vi "filter_peaks.vi"(8 "Correlation cluster":T3, 9 "Filter peak cluster":T2, 10 "Zero out":bool, 11 "Run Mode":bool) -> (0 "Blinking":bool, 1 "status":T1(ring), 3 "Filter peak output":T2)   [LabVIEW 2015]
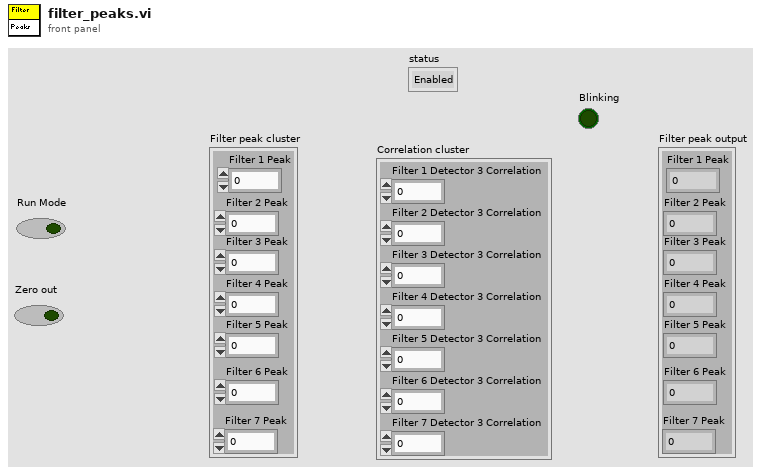
[diagram p1: front panel]
types:
  T1 = enum8{"Enabled", "Disabled", "Disabled and Grayed Out"}
  T2 = cluster{"Filter 1 Peak":i32, "Filter 2 Peak":i32, "Filter 3 Peak":i32, "Filter 4 Peak":i32, "Filter 5 Peak":i32, "Filter 6 Peak":i32, "Filter 7 Peak":i32}
  T3 = cluster{"Filter 1 Detector 3 Correlation":i32, "Filter 2 Detector 3 Correlation":i32, "Filter 3 Detector 3 Correlation":i32, "Filter 4 Detector 3 Correlation":i32, "Filter 5 Detector 3 Correlation":i32, "Filter 6 Detector 3 Correlation":i32, "Filter 7 Detector 3 Correlation":i32}
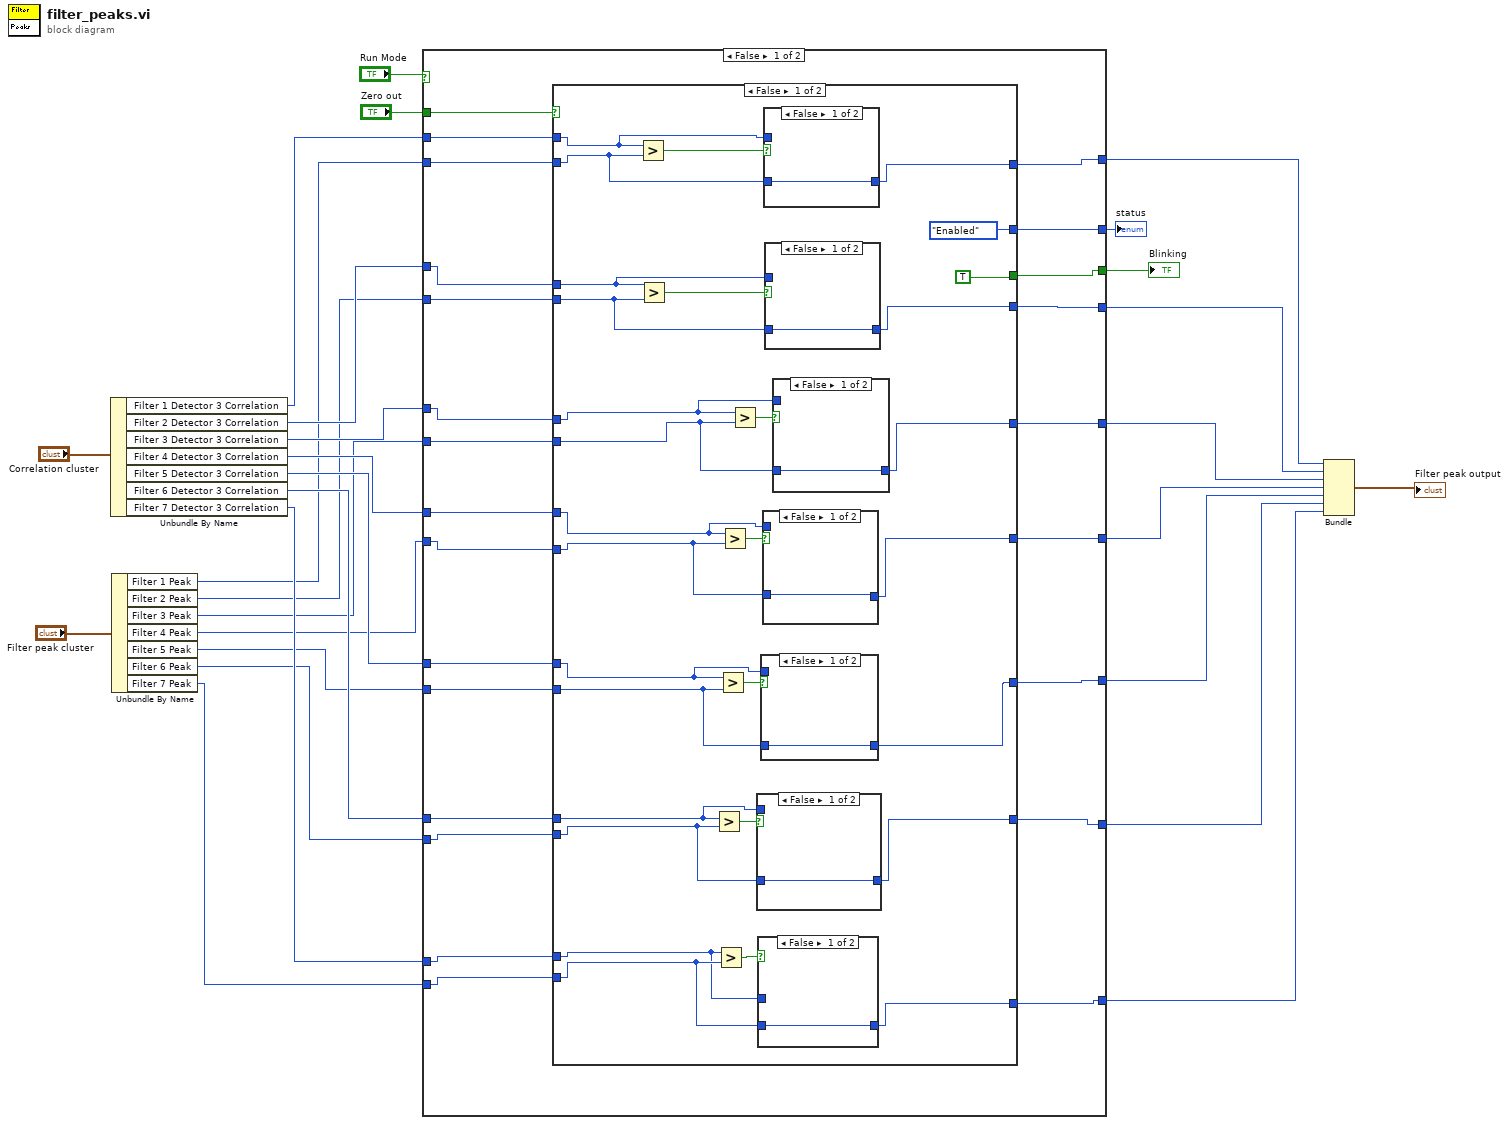
[diagram p0: block diagram]
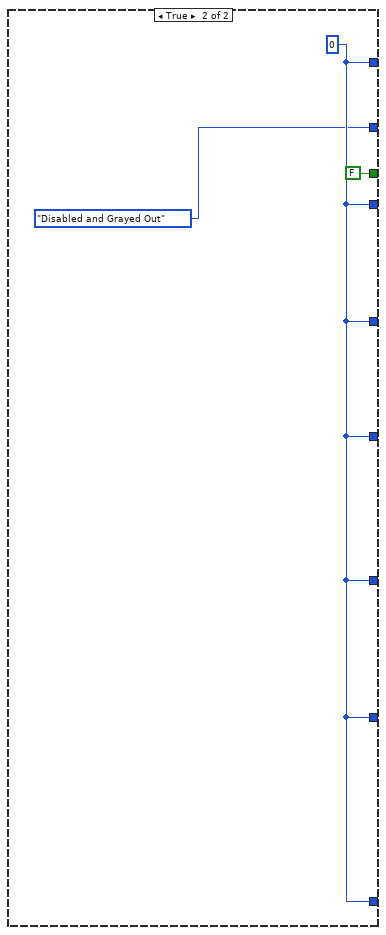
[diagram p9: hidden frame]
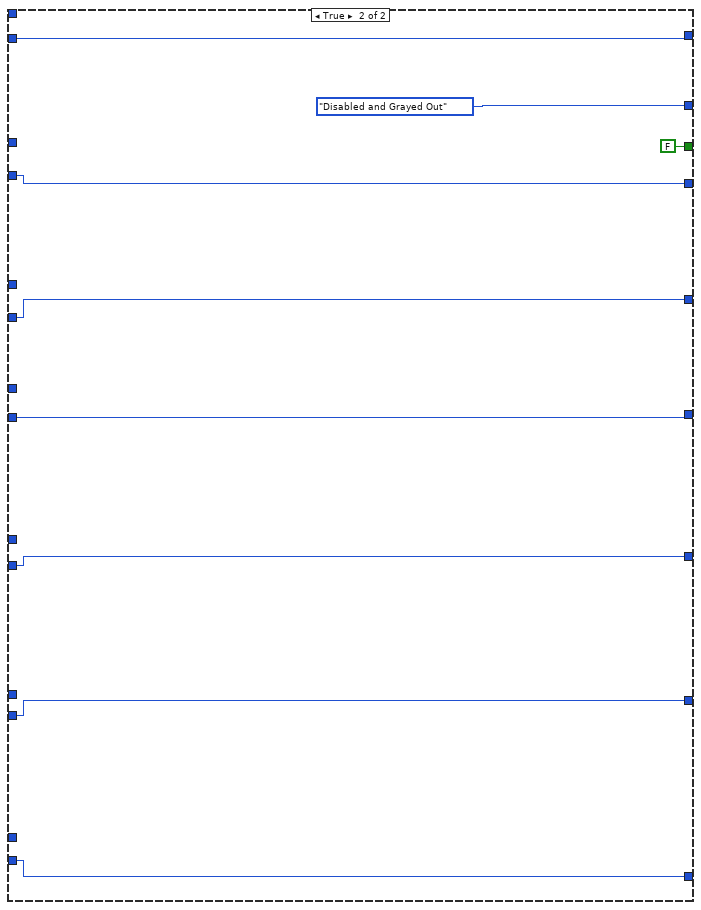
[diagram p10: hidden frame]
diagram:
  n1 = Unbundle By Name("Correlation cluster") -> ("Filter 1 Detector 3 Correlation"=w25:i32, "Filter 2 Detector 3 Correlation"=w24:i32, "Filter 3 Detector 3 Correlation"=w23:i32, "Filter 4 Detector 3 Correlation"=w22:i32, "Filter 5 Detector 3 Correlation"=w19:i32, "Filter 6 Detector 3 Correlation"=w21:i32, "Filter 7 Detector 3 Correlation"=w20:i32)
  n2 = Unbundle By Name("Filter peak cluster") -> ("Filter 1 Peak"=w17:i32, "Filter 2 Peak"=w16:i32, "Filter 3 Peak"=w15:i32, "Filter 4 Peak"=w14:i32, "Filter 5 Peak"=w13:i32, "Filter 6 Peak"=w12:i32, "Filter 7 Peak"=w11:i32)
  n3 = case shown="False" "Run Mode" {
    tunnel: [w52 w105] -> w8
    tunnel: [w51 w104] -> w7
    tunnel: [w50 w103] -> w6
    tunnel: [w49 w102] -> w5
    tunnel: [w48 w101] -> w4
    tunnel: [w47 w107] -> w10
    tunnel: [w46 w106] -> w9
    tunnel: "Zero out" -> [w45 _]
    tunnel: [w44 T1."Disabled and Grayed Out" ("Disabled")] -> w2
    tunnel: w25 -> [w43 _]
    tunnel: w24 -> [w42 _]
    tunnel: w23 -> [w41 _]
    tunnel: w22 -> [w40 _]
    tunnel: w21 -> [w38 _]
    tunnel: w20 -> [w37 _]
    tunnel: w19 -> [w39 _]
    tunnel: w17 -> [w36 w107]
    tunnel: w16 -> [w35 w106]
    tunnel: w15 -> [w34 w105]
    tunnel: w14 -> [w33 w104]
    tunnel: w13 -> [w32 w103]
    tunnel: w12 -> [w31 w102]
    tunnel: w11 -> [w30 w101]
    tunnel: [w29 FALSE] -> w1
    frame False {
      n4 = case shown="False" w45 {
        tunnel: [w67 w99] -> w52
        tunnel: [w64 w99] -> w51
        tunnel: [w61 w99] -> w50
        tunnel: [w58 w99] -> w49
        tunnel: [w55 w99] -> w48
        tunnel: [w72 w99] -> w47
        tunnel: [w70 w99] -> w46
        tunnel: [T1."Enabled" ("Disabled") T1."Disabled and Grayed Out" ("Disabled")] -> w44
        tunnel: w43 -> [w73 _]
        tunnel: w42 -> [w69 _]
        tunnel: w41 -> [w66 _]
        tunnel: w40 -> [w63 _]
        tunnel: w39 -> [w60 _]
        tunnel: w38 -> [w57 _]
        tunnel: w37 -> [w54 _]
        tunnel: w36 -> [w74 _]
        tunnel: w35 -> [w71 _]
        tunnel: w34 -> [w68 _]
        tunnel: w33 -> [w65 _]
        tunnel: w32 -> [w62 _]
        tunnel: w31 -> [w59 _]
        tunnel: w30 -> [w56 _]
        tunnel: [TRUE FALSE] -> w29
        frame False {
          n5 = Greater?(x=w73, y=w74) -> (0:w77:bool)
          n6 = Greater?(x=w69, y=w71) -> (0:w76:bool)
          n7 = Greater?(x=w57, y=w59) -> (0:w79:bool)
          n8 = Greater?(x=w54, y=w56) -> (0:w78:bool)
          n9 = Greater?(x=w60, y=w62) -> (0:w80:bool)
          n10 = Greater?(x=w63, y=w65) -> (0:w81:bool)
          n11 = Greater?(x=w66, y=w68) -> (0:w82:bool)
          n12 = case shown="False" w79 {
            tunnel: w59 -> [w89 _]
            tunnel: [w89 w90] -> w58
            tunnel: w57 -> [_ w90]
            frame False {
            }
            frame True {
            }
          }
          n13 = case shown="False" w78 {
            tunnel: w56 -> [w87 _]
            tunnel: [w87 w88] -> w55
            tunnel: w54 -> [_ w88]
            frame False {
            }
            frame True {
            }
          }
          n14 = case shown="False" w80 {
            tunnel: w62 -> [w91 _]
            tunnel: [w91 w92] -> w61
            tunnel: w60 -> [_ w92]
            frame False {
            }
            frame True {
            }
          }
          n15 = case shown="False" w81 {
            tunnel: w65 -> [w93 _]
            tunnel: [w93 w94] -> w64
            tunnel: w63 -> [_ w94]
            frame False {
            }
            frame True {
            }
          }
          n16 = case shown="False" w77 {
            tunnel: w74 -> [w85 _]
            tunnel: w73 -> [_ w86]
            tunnel: [w85 w86] -> w72
            frame False {
            }
            frame True {
            }
          }
          n17 = case shown="False" w76 {
            tunnel: w71 -> [w83 _]
            tunnel: [w83 w84] -> w70
            tunnel: w69 -> [_ w84]
            frame False {
            }
            frame True {
            }
          }
          n18 = case shown="False" w82 {
            tunnel: w68 -> [w95 _]
            tunnel: [w95 w96] -> w67
            tunnel: w66 -> [_ w96]
            frame False {
            }
            frame True {
            }
          }
        }
        frame True {
          w99 = 0
        }
      }
    }
    frame True {
    }
  }
  "status" <- w2
  "Blinking" <- w1
  n19 = Bundle("Filter 1 Peak"=w10, "Filter 2 Peak"=w9, "Filter 3 Peak"=w8, "Filter 4 Peak"=w7, "Filter 5 Peak"=w6, "Filter 6 Peak"=w5, "Filter 7 Peak"=w4) -> (→"Filter peak output":T2)  [unwired: 1 in]
